vi "put_element_by_name_from_binData.vi"(7 "little-endian?":bool, 8 "error in (no error)":errorcluster, 9 "value":variant, 10 "name":string, 11 "dataType in":variant) -> (0 "error out":errorcluster, 3 "data out":variant)   [LabVIEW 2015, in "BSON_convertors_Library.lvlib"]
doc: "Created by Artem Shevelev\nLabVIEW Portal profile: http://www.labviewportal.org/memberlist.php?mode=viewprofile&u=2340\ne-mail: artem.sh@gmail.com\nshevelev.pro"
uses:
  BSON_convertors_Library.lvlib
  typedefs/binaryData_cluster.ctl
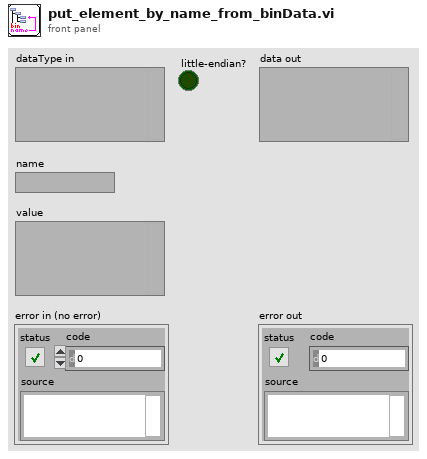
[diagram p1: front panel]
types:
  T1 = typedef "Type Descriptor Enumeration__ogtk.ctl" = enum8{"<Null>", "I8", "I16", "I32", "I64", "U8", "U16", "U32", "U64", "SGL", "DBL", "EXT", "CSG", "CDB", "CXT", "0x0F", "0x10", "0x11", "0x12", "0x13", "0x14", "Enum U8", "Enum U16", "Enum U32", "Enum U64", "SGL PQ", "DBL PQ", "EXT PQ", "CSG PQ", "CDB PQ", "CXT PQ", "0x1F", "0x20", "Boolean", "0x22", "0x23", "0x24", "0x25", "0x26", "0x27", "0x28", "0x29", "0x2A", "0x2B", "0x2C", "0x2D", "0x2E", "0x2F", "String", "0x31", "Path", "Pict", "0x34", "0x35", "0x36", "DAQ", "0x38", "0x39", "0x3A", "0x3B", "0x3C", "0x3D", "0x3E", "0x3F", "Array", "0x41", "0x42", "0x43", "0x44", "0x45", "0x46", "0x47", "0x48", "0x49", "0x4A", "0x4B", "0x4C", "0x4D", "0x4E", "0x4F", "Cluster", "0x51", "0x52", "Variant", "Waveform", "0x55", "0x56", "0x57", "0x58", "0x59", "0x5A", "0x5B", "0x5C", "0x5D", "0x5E", "Fixed Point", "0x60", "0x61", "0x62", "0x63", "0x64", "0x65", "0x66", "0x67", "0x68", "0x69", "0x6A", "0x6B", "0x6C", "0x6D", "0x6E", "0x6F", "Refnum", "0x71", "0x72", "Set Collection", "Map Collection"}
  T2 = typedef "BSON_convertors_Library.lvlib/binaryData_cluster.ctl" = cluster{"subType":u8, "byteArray":u8[]}
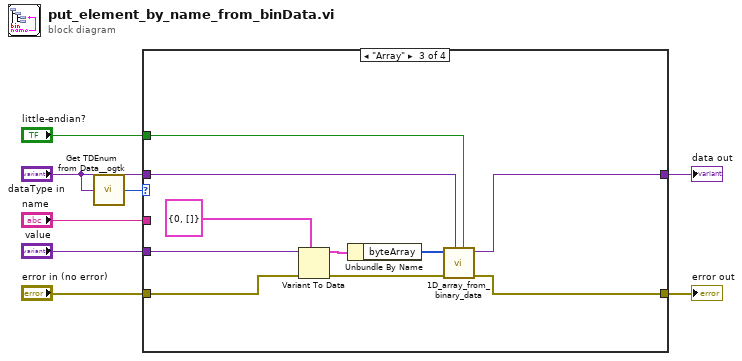
[diagram p0: block diagram]
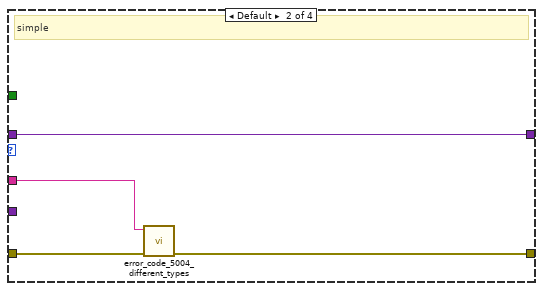
[diagram p3: hidden frame]
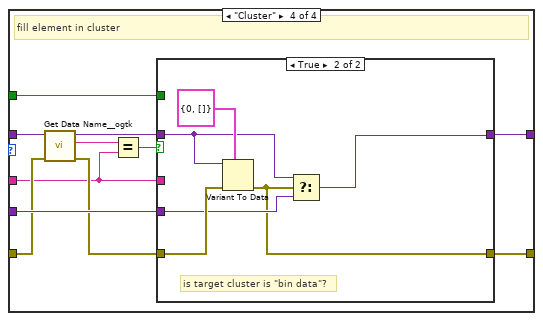
[diagram p4: hidden frame]
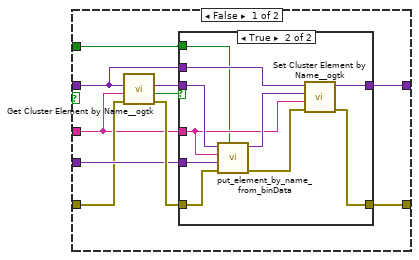
[diagram p5: hidden frame]
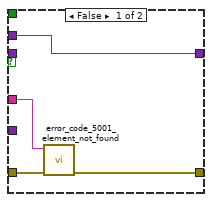
[diagram p6: hidden frame]
diagram:
  n1 = call <userlib>:"Get TDEnum from Data__ogtk.vi"("Data"="dataType in") -> ("Type Descriptor Enumeration"=w2:T1)  [unwired: 4 in]
  n2 = case shown="\"Array\"" w2 {
    tunnel: "dataType in" -> [w10 w11 w18 w32]
    tunnel: [w10 w11 w16 w34] -> w4
    tunnel: "value" -> [_ _ w24 w33]
    tunnel: "error in (no error)" -> [w9 w14 w23 w29]
    tunnel: [w9 w13 w15 w35] -> w7
    tunnel: "name" -> [_ w12 _ w27]
    tunnel: "little-endian?" -> [_ _ w17 w25]
    frame "<Null>" {
      # "error?\nor not?"
    }
    frame Default {
      # "simple"
      n3 = call "error_code_5004_different_types.vi"("error in (no error)"=w14, "name"=w12) -> ("error out"=w13:errorcluster)  [unwired: 9 in]
    }
    frame "Array" {
      n4 = Variant To Data(error in=w23, type=T2 {"subType"=0, "byteArray"=[]} ("binaryData"), Variant=w24) -> (data=w21:T2, error out=w19:errorcluster)
      n5 = Unbundle By Name(w21) -> ("byteArray"=w20:u8[])
      n6 = call "1D_array_from_binary_data.vi"("little-endian?"=w17, "inputArray(type)"=w18, "error in (no error)"=w19, "byteArray"=w20) -> ("error out"=w15:errorcluster, "dataArray"=w16:variant)  [unwired: 6 in]
    }
    frame "Cluster" {
      # "fill element in cluster"
      n7 = call <userlib>:"Get Data Name__ogtk.vi"("error in (no error)"=w29, "Data"=w32) -> ("error out"=w28:errorcluster, "Data Name"=w30:string, "Data dup"=w31:variant)  [unwired: 7 in]
      n8 = Equal?(x=w30, y=w27) -> (x = y?=w26:bool)
      n9 = case shown="True" w26 {
        tunnel: [w43 w60] -> w35
        tunnel: [w41 w62] -> w34
        tunnel: w33 -> [w40 w63]
        tunnel: w31 -> [w39 w61]
        tunnel: w28 -> [w38 w64]
        tunnel: w27 -> [w37 _]
        tunnel: w25 -> [w36 _]
        frame False {
          n10 = call <userlib>:"Get Cluster Element by Name__ogtk.vi"("error in (no error)"=w38, "Element Name"=w37, "Cluster"=w39) -> ("error out"=w44:errorcluster, "found?"=w45:bool, "VElement"=w42:variant)  [unwired: 6 in]
          n11 = case shown="True" w45 {
            tunnel: w37 -> [w49 w51]
            tunnel: w44 -> [w48 w55]
            tunnel: [w47 w57] -> w43
            tunnel: w42 -> [_ w53]
            tunnel: [w46 w58] -> w41
            tunnel: w39 -> [w46 w59]
            tunnel: w40 -> [_ w52]
            tunnel: w36 -> [_ w50]
            frame False {
              n12 = call "error_code_5001_element_not_found.vi"("error in (no error)"=w48, "name"=w49) -> ("error out"=w47:errorcluster)  [unwired: 9 in]
            }
            frame True {
              n13 = call "put_element_by_name_from_binData.vi"("little-endian?"=w50, "error in (no error)"=w55, "value"=w52, "name"=w51, "dataType in"=w53) -> ("error out"=w54:errorcluster, "data out"=w56:variant)  [unwired: 5 in]
              n14 = call <userlib>:"Set Cluster Element by Name__ogtk.vi"("error in (no error)"=w54, "Element Name (\"\": New Element Data Name)"=w51, "New Element Value"=w56, "Cluster"=w59) -> ("error out"=w57:errorcluster, "VCluster out"=w58:variant)  [unwired: 5 in, 1 out]
            }
          }
        }
        frame True {
          # "is target cluster is \"bin data\"?"
          n15 = Variant To Data(error in=w64, type=T2 {"subType"=0, "byteArray"=[]} ("binaryData"), Variant=w61) -> (error out=w60:errorcluster)  [unwired: 1 out]
          n16 = Select(t=w61, s=w60, f=w63) -> (s? t:f=w62:variant)
        }
      }
    }
  }
  "error out" <- w7
  "data out" <- w4
